vi "140116-Bilinear_interpolation.vi"(1 "multiplier":i32, 2 "Array":dbl[][](array[numeric])) -> (0 "10x Bilinear interpolation":dbl[][](graph))   [LabVIEW 2012]
uses:
  <vilib>/Analysis/1siggen.llb/Ramp Pattern by Samples.vi
  <vilib>/Analysis/NI_AALBase.lvlib
panel:
  out "Ramp Pattern":dbl[](array[numeric])
  out "original array":dbl[][](graph)
  # "http://forums.ni.com/ni/board/message?board.id=170&message.id=149301#M149301"
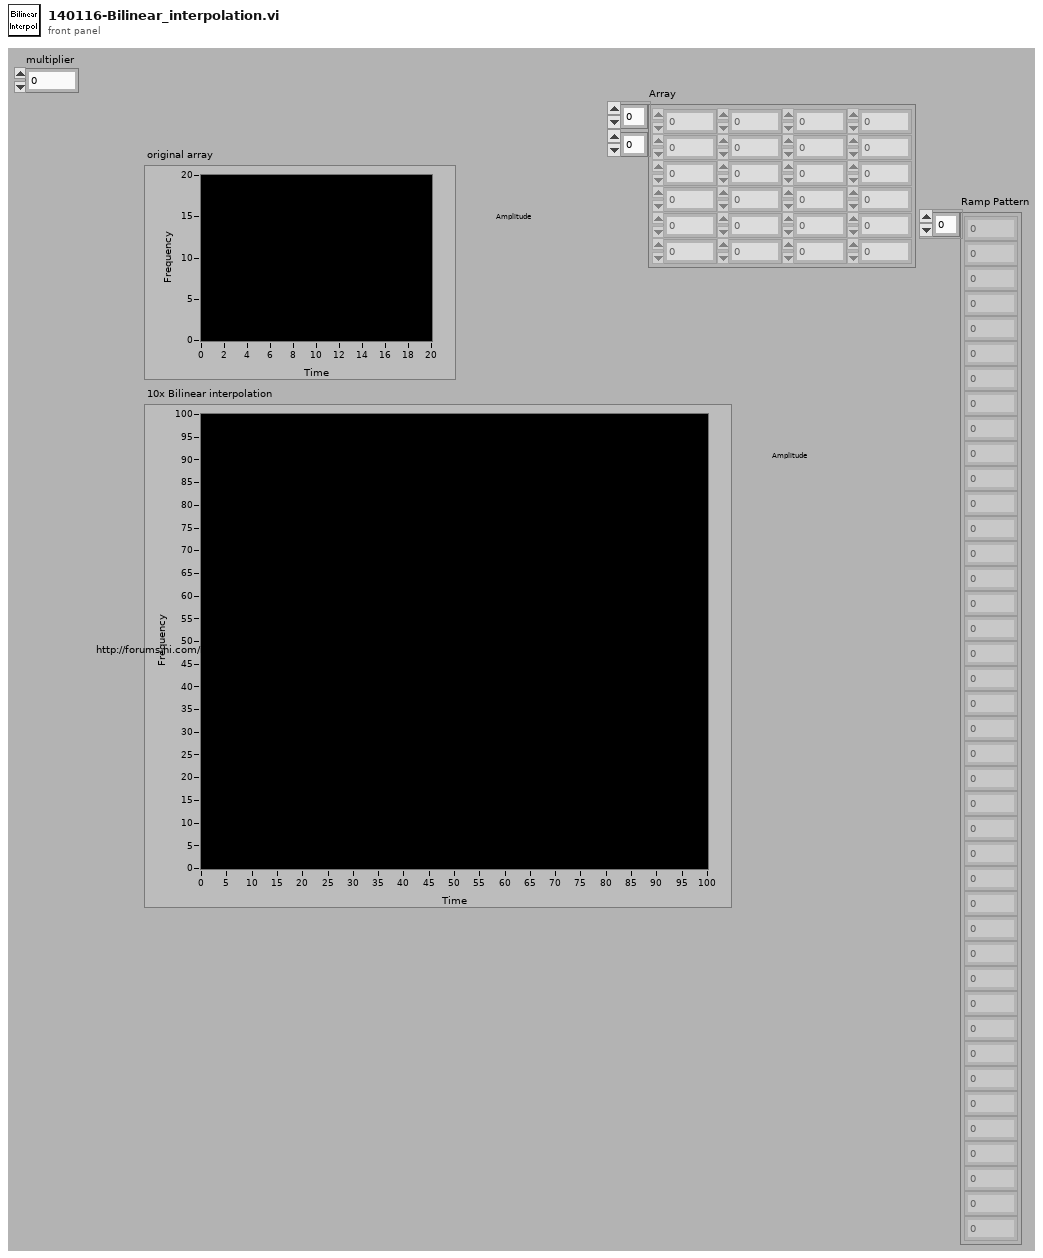
[diagram p1: front panel]
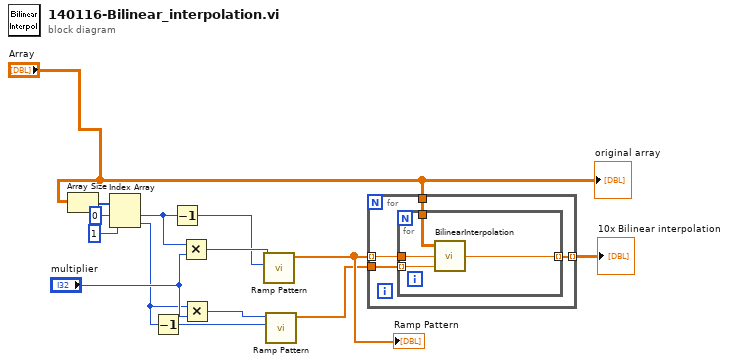
[diagram p0: block diagram]
diagram:
  n1 = Array Size(array="Array") -> (size(s)=w11:i32[])
  n2 = Index Array(array=w11, index #1=0 ("index"), index #2=1 ("index")) -> (element #1=w8:i32, element #2=w3:i32)
  n3 = Decrement(x=w3) -> (x-1=w2:i32)
  n4 = Decrement(x=w8) -> (x-1=w4:i32)
  n5 = Multiply(x=w8, y="multiplier") -> (x*y=w6:i32)
  n6 = Multiply(x=w3, y="multiplier") -> (x*y=w5:i32)
  n7 = call-poly <vilib>:"Ramp Pattern.vi"("end"=w4, "samples"=w6) -> ("Ramp Pattern"=w13:dbl[])  [unwired: 8 in, 1 out]
  "Ramp Pattern" <- w13
  n8 = call-poly <vilib>:"Ramp Pattern.vi"("end"=w2, "samples"=w5) -> ("Ramp Pattern"=w12:dbl[])  [unwired: 8 in, 1 out]
  n9 = for {
    tunnel: "Array" -> [w18]
    tunnel: w13 -> [w17] mode=indexing
    tunnel: w12 -> [w16]
    tunnel: [w15] -> w14 mode=indexing
    n10 = for {
      tunnel: w18 -> [w22]
      tunnel: w17 -> [w21]
      tunnel: w16 -> [w20] mode=indexing
      tunnel: [w19] -> w15 mode=indexing
      n11 = call "BilinearInterpolation.vi"("Column Index"=w20, "Row Index"=w21, "Array"=w22) -> ("Bilinear Interpolated Value"=w19:dbl)
    }
  }
  "10x Bilinear interpolation" <- w14
  "original array" <- "Array"
